vi "Shoot SSS.vi"(10 "Shoot Actuator Values In":T1) -> (2 "Shoot Actuator Values Out":T1)   [LabVIEW 2015]
uses:
  Shoot Actuator Values.ctl
  <vilib>/Rock Robotics/WPI/Solenoid/WPI_SolenoidValue.ctl
  Global Variables/refnum names.vi
  Global Variables/Settings.vi
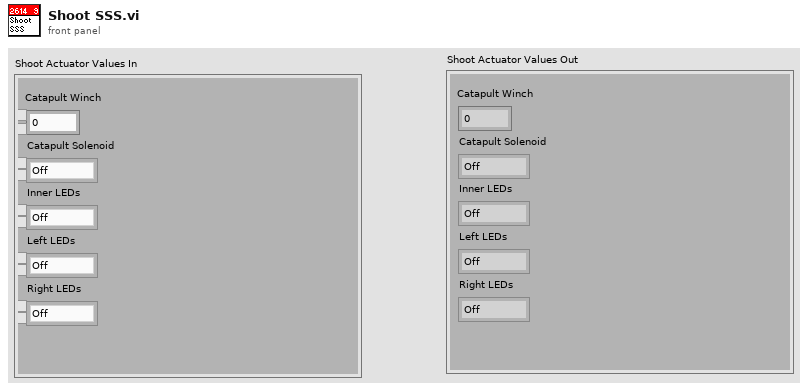
[diagram p1: front panel]
types:
  T1 = typedef "Shoot Actuator Values.ctl" = cluster{"Catapult Winch":dbl, "Catapult Solenoid":T2, "Inner LEDs":T2, "Left LEDs":T2, "Right LEDs":T2}
  T2 = typedef "WPI_SolenoidValue.ctl" = enum16{"Off", "On", "Forward", "Reverse"}
  T3 = typedef "WPI_MotorControlDeviceRef.ctl" = cluster{"DeviceStatus":errorcluster, "Type":T4, "PWM":cluster{"PWM Channel":T5, "DeadBand":T6}, "CAN":cluster{"Device Number":u8, "Control Mode":T7, "Semaphore":T8, "Max Vout":dbl, "TalonSRX Control Mode":T9}, "Invert":bool}
  T4 = typedef "WPI_MotorControlType.ctl" = enum16{"PWM", "CAN", "CANTalonSRX"}
  T5 = typedef "FPGA_DIOPWMChannel.ctl" = enum8{"PWM 0", "PWM 1", "PWM 2", "PWM 3", "PWM 4", "PWM 5", "PWM 6", "PWM 7", "PWM 8", "PWM 9", "PWM MXP 0", "PWM MXP 1", "PWM MXP 2", "PWM MXP 3", "PWM MXP 4", "PWM MXP 5", "PWM MXP 6", "PWM MXP 7", "PWM MXP 8", "PWM MXP 9", "Invalid"}
  T6 = typedef "WPI_PWMDeadband.ctl" = cluster{"Name":string, "maxPositivePwm":i32, "minPositivePwm":i32, "centerPwm":i32, "maxNegativePwm":i32, "minNegativePwm":i32, "angularRange":u16}
  T7 = typedef "WPI_CANJaguar_ControlMode.ctl" = enum8{"Percent VBus", "Current", "Speed", "Position", "Voltage"}
  T8 = typedef "Semaphore RefNum" = refnum<k1>
  T9 = typedef "WPI_CANTalonSRX_APIControlMode.ctl" = enum8{"Percent VBus", "Speed", "Position", "Slave", "Unchanged / Invalid", "Voltage Compensation", "Current", "Motion Profile"}
  T10 = typedef "WPI_CANTalonSRX_GlobalStatus.ctl" = cluster{"Applied Throttle":dbl, "Module Enabled":bool, "CAN Error":errorcluster, "Closed Loop Error":dbl, "Forward Limit Switch Closed":bool, "Reverse Limit Switch Closed":bool, "Sensor Position":dbl, "Sensor Velocity":dbl, "Current":dbl, "Sticky Fault - Over Temp":bool, "Sticky Fault - Under Voltage":bool, "Sticky Fault - Forward Limit":bool, "Sticky Fault - Reverse Limit":bool, "Sticky Fault - Forward Soft Limit":bool, "Sticky Fault - Reverse Soft Limit":bool, "Brake is Enabled":bool, "Encoder Position":dbl, "Encoder Velocity":dbl, "Encoder Index Count":dbl, "Encoder A Pin State":bool, "Encoder B Pin State":bool, "Encoder Index Pin State":bool, "Analog In":dbl, "Analog In Velocity":dbl, "Temperature (C)":dbl, "Battery Voltage":dbl, "Control 5 Is Supported":bool, "Current Profile Slot Select":dbl, "Pos Div 8":bool, "Vel Div 4":bool, "Pulse Width Position":i32, "Pulse Width Velocity":i32, "Pulse Width Rise To Rise (us)":i32, "Pulse Width Rise To Fall (us)":i32, "Mot Prof Active Is Under Run":bool, "Mot Prof Active Has Under Run":bool, "Mot Prof Active Is Last":bool, "Mot Prof Active Velocity Only":bool, "Mot Prof Active Is Valid":bool, "Mot Prof Buffer Is Full":bool, "Mot Prof Active Profile Slot Select":i32, "Mot Prof NextID":i32, "Mot Prof Count":i32, "Mot Prof Active Velocity":dbl, "Mot Prof Active Position":dbl, "Mot Prof Output Enable":i32}
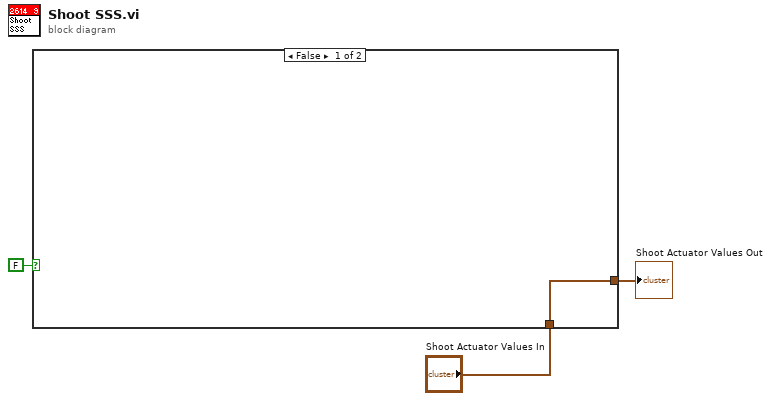
[diagram p0: block diagram]
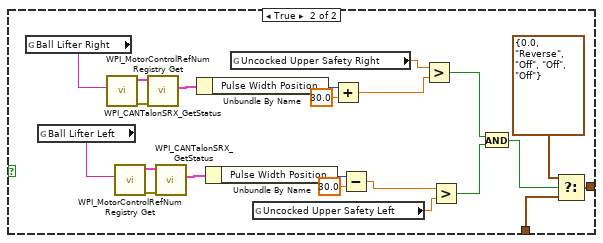
[diagram p2: hidden frame]
diagram:
  n1 = case shown="False" FALSE {
    tunnel: "Shoot Actuator Values In" -> [w4 w26]
    tunnel: [w4 w25] -> w2
    frame False {
    }
    frame True {
      n2 = global read "refnum names.vi" "Ball Lifter Right"() -> (w18:string)
      n3 = global read "refnum names.vi" "Ball Lifter Left"() -> (w17:string)
      n4 = call <vilib>:"WPI_MotorControlRefNum Registry Get.vi"("refnum name"=w18) -> ("error out"=w20:errorcluster, "MotorControlDevRef"=w19:T3)  [unwired: 9 in]
      n5 = call <vilib>:"WPI_MotorControlRefNum Registry Get.vi"("refnum name"=w17) -> ("error out"=w15:errorcluster, "MotorControlDevRef"=w16:T3)  [unwired: 9 in]
      n6 = call <vilib>:"WPI_CANTalonSRX_GetStatus.vi"("error in (no error)"=w20, "CAN Talon SRX Ref"=w19) -> ("Talon SRX Status"=w22:T10)  [unwired: 7 in, 2 out]
      n7 = call <vilib>:"WPI_CANTalonSRX_GetStatus.vi"("error in (no error)"=w15, "CAN Talon SRX Ref"=w16) -> ("Talon SRX Status"=w14:T10)  [unwired: 7 in, 2 out]
      n8 = Unbundle By Name(w22) -> ("Pulse Width Position"=w24:i32)
      n9 = Unbundle By Name(w14) -> ("Pulse Width Position"=w12:i32)
      n10 = global read "Settings.vi" "Uncocked Upper Safety Right"() -> (w6:dbl)
      n11 = global read "Settings.vi" "Uncocked Upper Safety Left"() -> (w5:dbl)
      n12 = Add(x=w24, y=30.0) -> (x+y=w21:dbl)
      n13 = Subtract(x=w12, y=30.0) -> (x-y=w11:dbl)
      n14 = Greater?(x=w6, y=w21) -> (0:w10:bool)
      n15 = Greater?(x=w11, y=w5) -> (0:w9:bool)
      n16 = And(x=w10, y=w9) -> (x .and. y?=w8:bool)
      n17 = Select(t=T1 {"Catapult Winch"=0.0, "Catapult Solenoid"=enum."Reverse", "Inner LEDs"=enum."Off", "Left LEDs"=enum."Off", "Right LEDs"=enum."Off"}, s=w8, f=w26) -> (s? t:f=w25:T1)
    }
  }
  "Shoot Actuator Values Out" <- w2
